vi "Set Out IPS120.vi"(8 "Error In":errorcluster, 10 "Set output":T1={"Set point"=0.0, "Sweep rate"=0.1, "Sweep action"=enum."To set point"}, 11 "VISA resource name":refnum<visa-resource-name>) -> (0 "Error Out":errorcluster, 3 "VISA resource name out":refnum<visa-resource-name>)   [LabVIEW 2018]
uses:
  Controls/Set Output.ctl
  Controls/Sweep Action.ctl
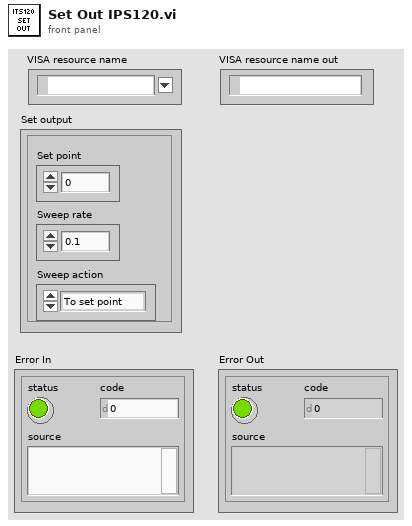
[diagram p1: front panel]
types:
  T1 = typedef "Set Output.ctl" = cluster{"Set point":dbl, "Sweep rate":dbl, "Sweep action":T2}
  T2 = typedef "Sweep Action.ctl" = enum16{"Hold", "To set point", "To zero", "Clamp"}
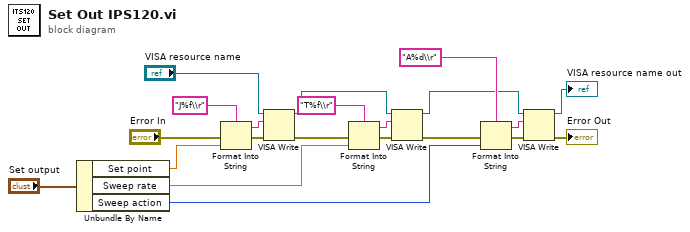
[diagram p0: block diagram]
diagram:
  n1 = Unbundle By Name("Set output") -> ("Set point"=w19:dbl, "Sweep rate"=w11:dbl, "Sweep action"=w4:T2)
  n2 = Format Into String(format string="J%f\\r", error in="Error In", w19) -> (resulting string=w15:string, error out=w17:errorcluster)  [unwired: 1 in]
  n3 = VISA Write(VISA resource name="VISA resource name", write buffer=w15, error in (no error)=w17) -> (VISA resource name out=w9:refnum<visa-resource-name>, error out=w10:errorcluster)  [unwired: 1 out]
  n4 = Format Into String(format string="T%f\\r", error in=w10, w11) -> (resulting string=w14:string, error out=w13:errorcluster)  [unwired: 1 in]
  n5 = VISA Write(VISA resource name=w9, write buffer=w14, error in (no error)=w13) -> (VISA resource name out=w3:refnum<visa-resource-name>, error out=w5:errorcluster)  [unwired: 1 out]
  n6 = Format Into String(format string="A%d\\r", error in=w5, w4) -> (resulting string=w6:string, error out=w7:errorcluster)  [unwired: 1 in]
  n7 = VISA Write(VISA resource name=w3, write buffer=w6, error in (no error)=w7) -> (VISA resource name out=→"VISA resource name out":refnum<visa-resource-name>, error out=→"Error Out":errorcluster)  [unwired: 1 out]
